vi "Read Attributes.vi"(11 "Return String Msg":refnum<class "Return String Msg.lvclass">) -> (2 "Payload":cluster{"String":string})   [LabVIEW 2018, in "EMS Generic Actor.lvlib" / "Return String Msg.lvclass"]
uses:
  Return String Msg.lvclass
  Return String Msg.lvclass/Return String Msg.ctl
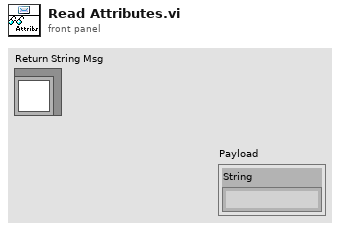
[diagram p1: front panel]
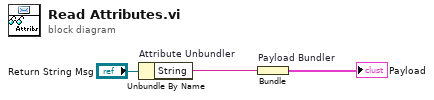
[diagram p0: block diagram]
diagram:
  n1 = Unbundle By Name "Attribute Unbundler"("Return String Msg") -> ("String"=w1:string)
  n2 = Bundle "Payload Bundler"("String"=w1) -> (→"Payload":cluster{"String":string})  [unwired: 1 in]
